vi "Set Temp Setpoint--Method.vi"(8 "error in (no error)":errorcluster, 10 "Temp Setpoint Data":T1, 11 "Simulated Thermal Process Controller in":refnum<class "Simulated Thermal Process Controller.lvclass">) -> (0 "error out":errorcluster, 3 "Simulated Thermal Process Controller out":refnum<class "Simulated Thermal Process Controller.lvclass">)   [LabVIEW 2024, in "Simulated Thermal Process Controller.lvclass"]
uses:
  Simulated Thermal Process Controller.lvclass
  Process Controller/Controls/Temp Data--Cluster.ctl
  Process Controller/Controls/Temperature Units--Enum.ctl
  Simulated Thermal Process Controller.lvclass/Simulated Thermal Process Controller.ctl
  Process Controller/_Thermal Process Controller.lvclass
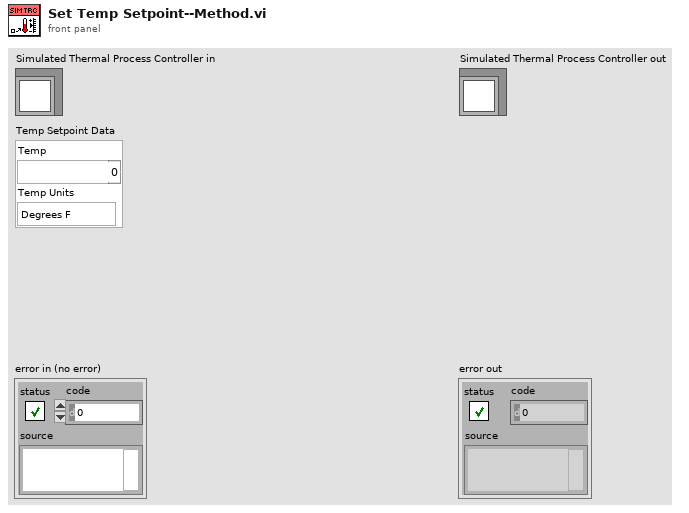
[diagram p1: front panel]
types:
  T1 = typedef "_Thermal Process Controller.lvclass/Temp Data--Cluster.ctl" = cluster{"Temp":dbl, "Temp Units":T2}
  T2 = typedef "_Thermal Process Controller.lvclass/Temperature Units--Enum.ctl" = enum16{"Degrees F", "Degrees C", "Degrees K"}
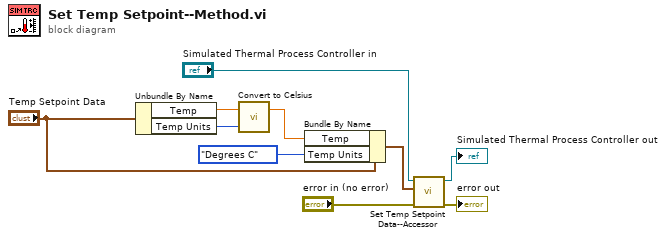
[diagram p0: block diagram]
diagram:
  n1 = Unbundle By Name("Temp Setpoint Data") -> ("Temp"=w2:dbl, "Temp Units"=w3:T2)
  n2 = call "Convert to Celsius.vi"("Temp In"=w2, "Temp Units"=w3) -> ("Temp Out"=w6:dbl)  [unwired: 3 in]
  n3 = Bundle By Name(cluster="Temp Setpoint Data", "Temp"=w6, "Temp Units"=Temperature_Units--Enum."Degrees C") -> (w1:T1)
  n4 = call "Set Temp Setpoint Data--Accessor.vi"("error in (no error)"="error in (no error)", "Temp Setpoint Data"=w1, "Simulated Thermal Process Controller in"="Simulated Thermal Process Controller in") -> ("error out"=→"error out":errorcluster, "Simulated Thermal Process Controller out"=→"Simulated Thermal Process Controller out":refnum<class "Simulated Thermal Process Controller.lvclass">)  [unwired: 7 in]
